vi "Update HTML File.vi"(10 "Data In":T1, 11 "Path":path) -> (3 "URL out":string)   [LabVIEW 2020, in "Pie Chart.xctl"]
uses:
  Pie Chart.xctl
  Data Pie Chart.ctl
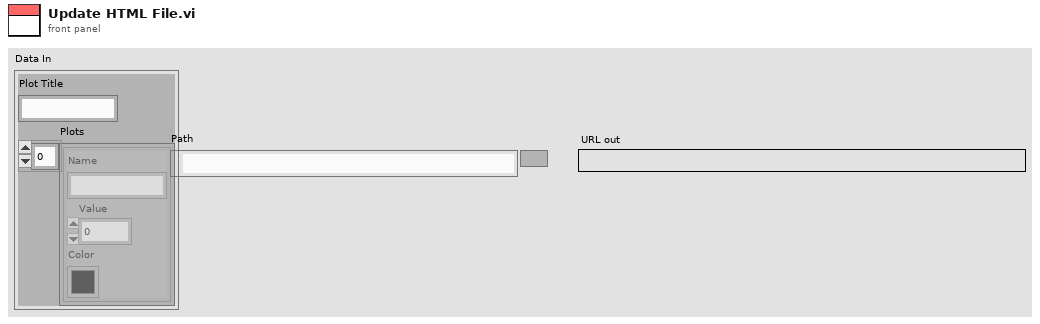
[diagram p1: front panel]
types:
  T1 = typedef "Pie Chart.xctl/Data Pie Chart.ctl" = cluster{"Plot Title":string, "Plots":cluster{"Name":string, "Value":dbl, "Color":u32}[]}
  T2 = enum16{"open", "replace", "create", "open or create", "replace or create", "replace or create with confirmation"}
  T3 = cluster{"Name":string, "Value":dbl, "Color":u32}[]
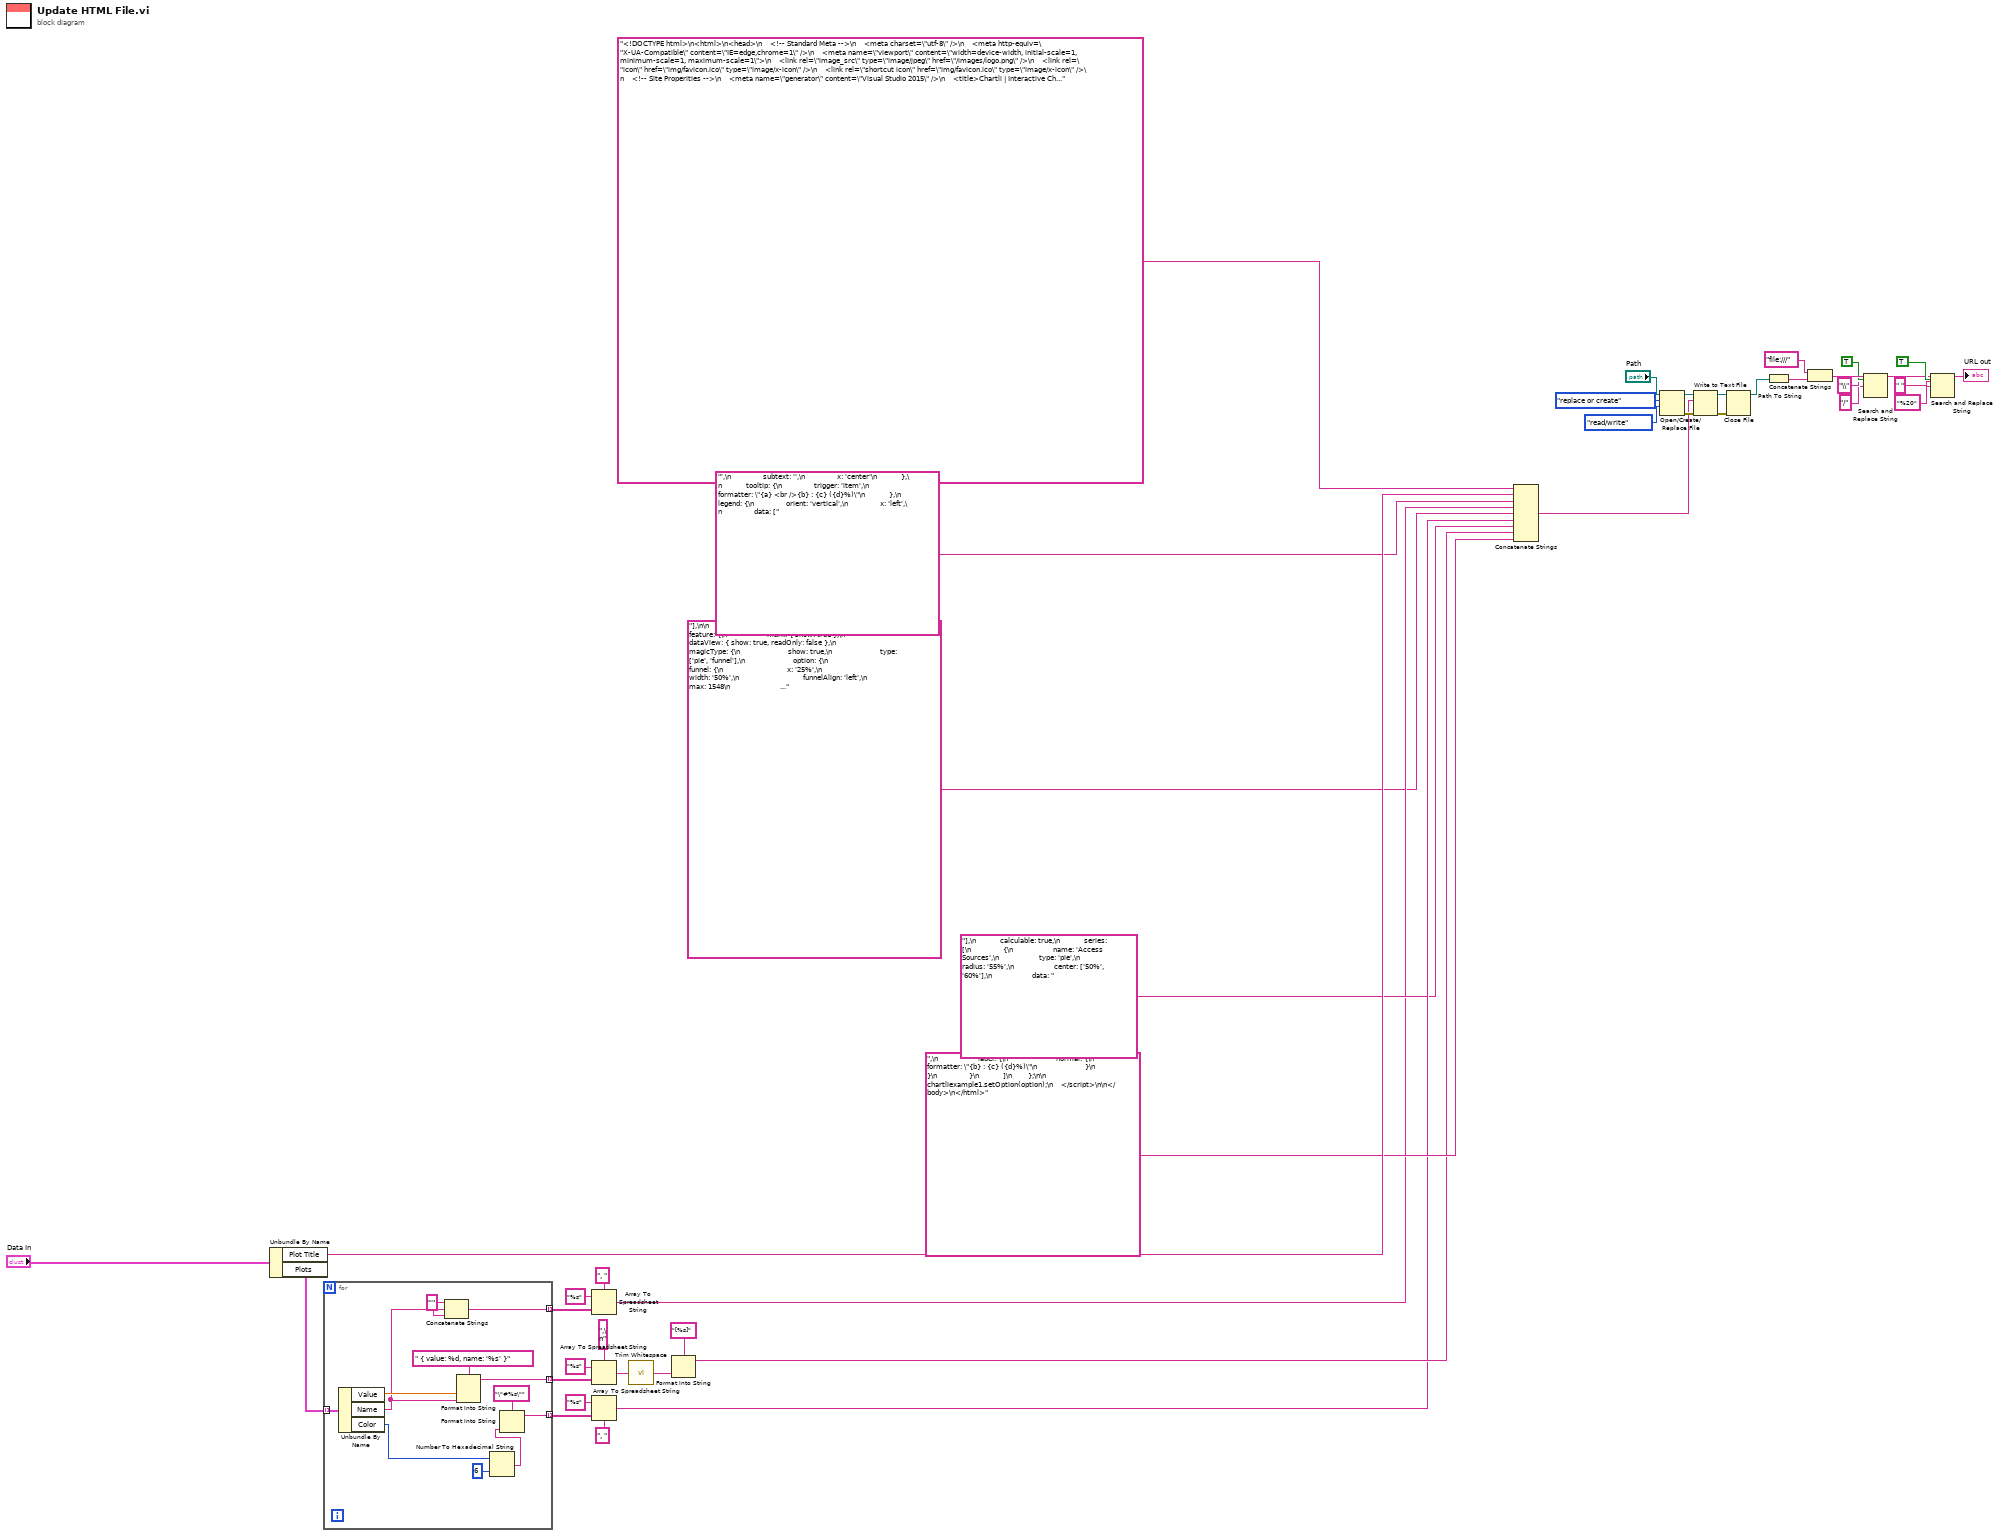
[diagram p0: block diagram]
diagram:
  n1 = Unbundle By Name("Data In") -> ("Plot Title"=w42:string, "Plots"=w38:T3)
  n2 = for {
    tunnel: w38 -> [w55] mode=indexing
    tunnel: [w52] -> w34 mode=indexing
    tunnel: [w50] -> w10 mode=indexing
    tunnel: [w47] -> w3 mode=indexing
    w48 = "'" ("string")
    n3 = Unbundle By Name(w55) -> ("Value"=w53:dbl, "Name"=w49:string, "Color"=w44:u32)
    n4 = Concatenate Strings(w48, w49, w48) -> (w47:string)
    n5 = Format Into String(format string=" { value: %d, name: '%s' }", w53, w49) -> (resulting string=w52:string)  [unwired: 2 in, 1 out]
    n6 = Number To Hexadecimal String(1:i16 6 ("width (-)"), 2:w44) -> (0:w45:string)
    n7 = Format Into String(format string="\"#%s\"", w45) -> (resulting string=w50:string)  [unwired: 2 in, 1 out]
  }
  n8 = Array To Spreadsheet String(delimiter (Tab)=", ", array=w3, 3:"%s" ("format string")) -> (spreadsheet string=w2:string)
  n9 = Array To Spreadsheet String(delimiter (Tab)=",\n", array=w34, 3:"%s" ("format string")) -> (spreadsheet string=w36:string)
  n10 = Array To Spreadsheet String(delimiter (Tab)=", ", array=w10, 3:"%s" ("format string")) -> (spreadsheet string=w7:string)
  n11 = call <vilib>:"Trim Whitespace.vi"("string"=w36) -> ("trimmed string"=w35:string)  [unwired: 1 in]
  n12 = Format Into String(format string="[%s]", w35) -> (resulting string=w8:string)  [unwired: 2 in, 1 out]
  n13 = Concatenate Strings("<!DOCTYPE html>\n<html>\n<head>\n    <!-- Standard Meta -->\n    <meta charset=\"utf-8\" />\n    <meta http-equiv=\"X-UA-Compatible\" content=\"IE=edge,chrome=1\" />\n    <meta name=\"viewport\" content=\"width=device-width, initial-scale=1, minimum-scale=1, maximum-scale=1\">\n    <link rel=\"image_src\" type=\"image/jpeg\" href=\"/images/logo.png\" />\n    <link rel=\"icon\" href=\"img/favicon.ico\" type=\"image/x-icon\" />\n    <link rel=\"shortcut icon\" href=\"img/favicon.ico\" type=\"image/x-icon\" />\n    <!-- Site Properities -->\n    <meta name=\"generator\" content=\"Visual Studio 2015\" />\n    <title>Chartli | Interactive Chart</title>\n    <meta name=\"description\" content=\"Chartli Interactive Chart\" />\n    <meta name=\"keywords\" content=\"html5,chart,ui, library, framework, javascript,jquery,graphic,interactive\" />\n    <link href=\"css/semantic.css\" rel=\"stylesheet\" />\n    <link href=\"css/demo.css\" rel=\"stylesheet\" />\n</head>\n<body>\n\n    <div id=\"pieChart1\" style=\"height:100%;\"></div>\n\n    <script src=\"js/jquery-2.1.4.min.js\"></script>\n    <script src=\"js/chartli.js\"></script>\n    <script type=\"text/javascript\">\n\n        var chartliexample1 = echarts.init(document.getElementById('pieChart1'));\n\n        option = {\n            backgroundColor: '#FFFFF',\n\n            title: {\n                text: '", w42, "',\n                subtext: '',\n                x: 'center'\n            },\n            tooltip: {\n                trigger: 'item',\n                formatter: \"{a} <br />{b} : {c} ({d}%)\"\n            },\n            legend: {\n                orient: 'vertical',\n                x: 'left',\n                data: [", w2, "],\n\n            },\n            toolbox: {\n                show: true,\n                feature: {\n                    mark: { show: true },\n                    dataView: { show: true, readOnly: false },\n                    magicType: {\n                        show: true,\n                        type: ['pie', 'funnel'],\n                        option: {\n                            funnel: {\n                                x: '25%',\n                                width: '50%',\n                                funnelAlign: 'left',\n                                max: 1548\n                            }\n                        }\n                    },\n                    restore: { show: true },\n                    saveAsImage: { show: true }\n                }\n            },\n            color: [", w7, "],\n            calculable: true,\n            series: [\n                {\n                    name: 'Access Sources',\n                    type: 'pie',\n                    radius: '55%',\n                    center: ['50%', '60%'],\n                    data: ", w8, ",\n                    label: {\n                        normal: {\n                            formatter: \"{b} : {c} ({d}%)\"\n                        }\n                    }\n                }\n            ]\n        };\n\n        chartliexample1.setOption(option);\n    </script>\n\n</body>\n</html>") -> (w12:string)
  n14 = Open/Create/Replace File(file path (use dialog)="Path", operation (0:open)=T2."replace or create", access (0:read/write)=enum16{"read/write", "read-only", "write-only"}."read/write") -> (refnum out=w29:refnum<file>, error out=w23:errorcluster)  [unwired: 3 in, 1 out]
  n15 = Write to Text File(file (use dialog)=w29, text=w12, error in=w23) -> (refnum out=w27:refnum<file>, error out=w22:errorcluster)  [unwired: 1 in, 1 out]
  n16 = Close File(refnum=w27, error in=w22) -> (path=w24:path)  [unwired: 1 out]
  n17 = Path To String(path=w24) -> (string=w26:string)
  n18 = Concatenate Strings("file:///" ("string"), w26) -> (w21:string)
  n19 = Search and Replace String(replace all?=TRUE ("replace all? (F)"), input string=w21, search string="\\", replace string="/" ("replace string (\"\")")) -> (result string=w14:string)  [unwired: 4 in, 3 out]
  n20 = Search and Replace String(replace all?=TRUE ("replace all? (F)"), input string=w14, search string=" ", replace string="%20" ("replace string (\"\")")) -> (result string=→"URL out":string)  [unwired: 4 in, 3 out]
